vi "initializer_highlight_validation.vi"(9 "validationErrors":string, 10 "Parameters Tree":refnum<vi>) -> ()   [LabVIEW 2019]
panel:
  # "*******************************************************************\nBiogas Plant Control\n\nAuthor: Paul Zügel\nGCSC-Frankfurt am Main 2020\n\n*******************************************************************"
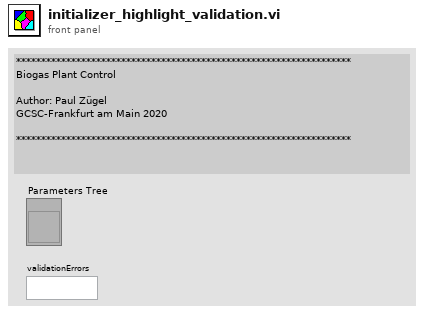
[diagram p1: front panel]
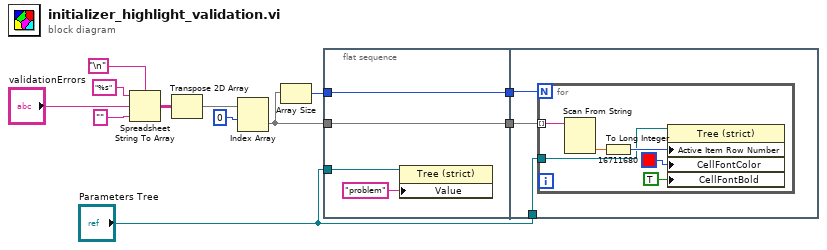
[diagram p0: block diagram]
diagram:
  n1 = Spreadsheet String To Array(delimiter (Tab)="\n", format string="%s", spreadsheet string="validationErrors", array type (2D Dbl)="") -> (array=w4:string[][])
  n2 = Transpose 2D Array(2D array=w4) -> (transposed array=w5:string[][])
  n3 = Index Array(array=w5, index (row)=0) -> (element=w10:string[])  [unwired: 1 in]
  n4 = Array Size(array=w10) -> (size(s)=w9:i32)
  n5 = flat-sequence {
    tunnel: w10 -> [w15]
    tunnel: w9 -> [w16]
    tunnel: [w16] -> w12
    tunnel: [w15] -> w11
    tunnel: "Parameters Tree" -> [w14]
    tunnel: w12 -> [w19]
    tunnel: w11 -> [w18]
    tunnel: "Parameters Tree" -> [w17]
    frame #0 {
      n6 = property class="Tree (strict)"(reference=w14, "Value"="problem" ("Active Item:Tag")) -> ()  [unwired: 1 in, 2 out]
    }
    frame #1 {
      n7 = for {
        N: w19 -> [_]
        tunnel: w18 -> [w24] mode=indexing
        tunnel: w17 -> [w21]
        n8 = Scan From String(input string=w24) -> (output 1=w23:dbl)  [unwired: 4 in, 3 out]
        n9 = To Long Integer(number=w23) -> (32bit integer=w22:i32)
        n10 = property on="Property Node" class="Tree (strict)"(reference=w21, "Active Item Row Number"=w22, "CellFontColor"=u32 16711680, "CellFontBold"=TRUE ("Active Cell:Cell Font:Bold")) -> ()  [unwired: 1 in, 2 out]
      }
    }
  }
